vi "Continuous.vi"(8 "error in":errorcluster, 10 "Continuous Measurement (true)":bool=TRUE, 11 "VISA resource name":refnum<visa-resource-name>) -> (0 "error out":errorcluster, 3 "VISA resource name out":refnum<visa-resource-name>)   [LabVIEW 2017, in "Andeen-Hagerling 2700.lvlib"]
doc: "This VI initiates or halts continuous capacitance measurement by the bridge."
uses:
  Andeen-Hagerling 2700.lvlib
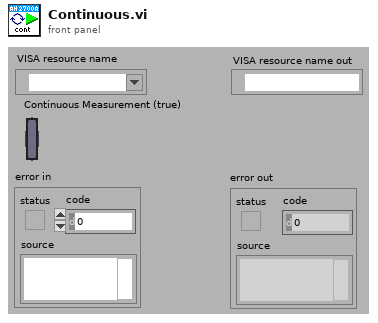
[diagram p1: front panel]
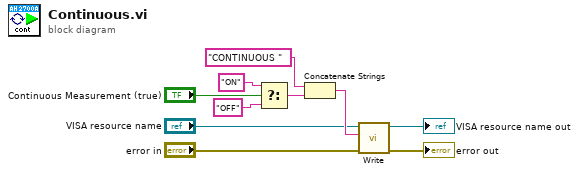
[diagram p0: block diagram]
diagram:
  n1 = Select(t="ON", s="Continuous Measurement (true)", f="OFF") -> (s? t:f=w4:string)
  n2 = Concatenate Strings("CONTINUOUS " ("command"), w4) -> (w3:string)
  n3 = call "Write.vi"("error in"="error in", "command"=w3, "VISA resource name"="VISA resource name") -> ("error out"=→"error out":errorcluster, "VISA resource name out"=→"VISA resource name out":refnum<visa-resource-name>)  [unwired: 7 in]
